vi "Pixy_COM-RIO.vi"() -> ()   [LabVIEW 2015]
uses:
  <vilib>/Analysis/baseanly.llb/Mean (DBL).vi
  <vilib>/Instr/_visa.llb/VISA Configure Serial Port (Instr).vi
  <vilib>/Analysis/NI_AALBase.lvlib
panel:
  in  "Debug?":bool
  out "Data display":string
  in  "Write Command?":bool
  in  "Command":string(combo)
  out "Area":dbl(graph)
  out "Height":i32
  out "Width":i32
  out "Y":i32
  out "X":i32
  out "Read error out":errorcluster
  out "Initialization error out":errorcluster
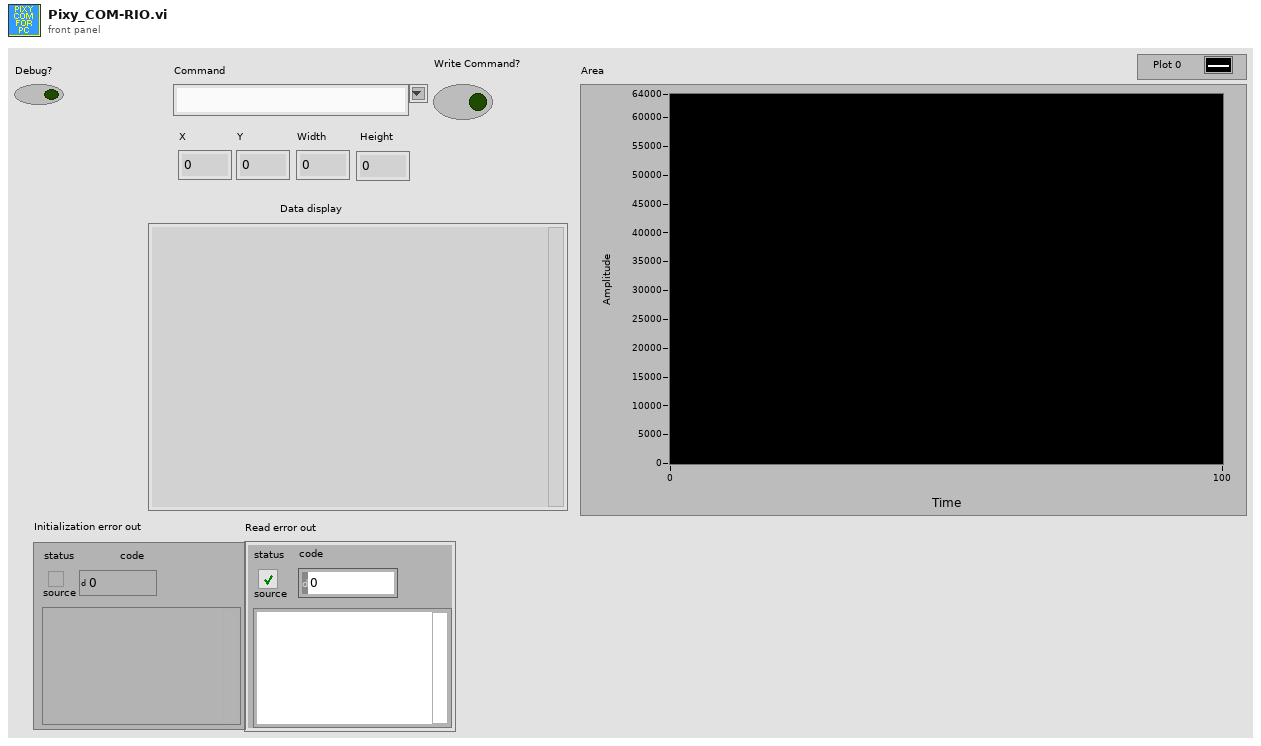
[diagram p1: front panel]
types:
  T1 = cluster{"buffer":string, "X":i32, "Y":i32, "Width":i32, "Height":i32, "Area":dbl}
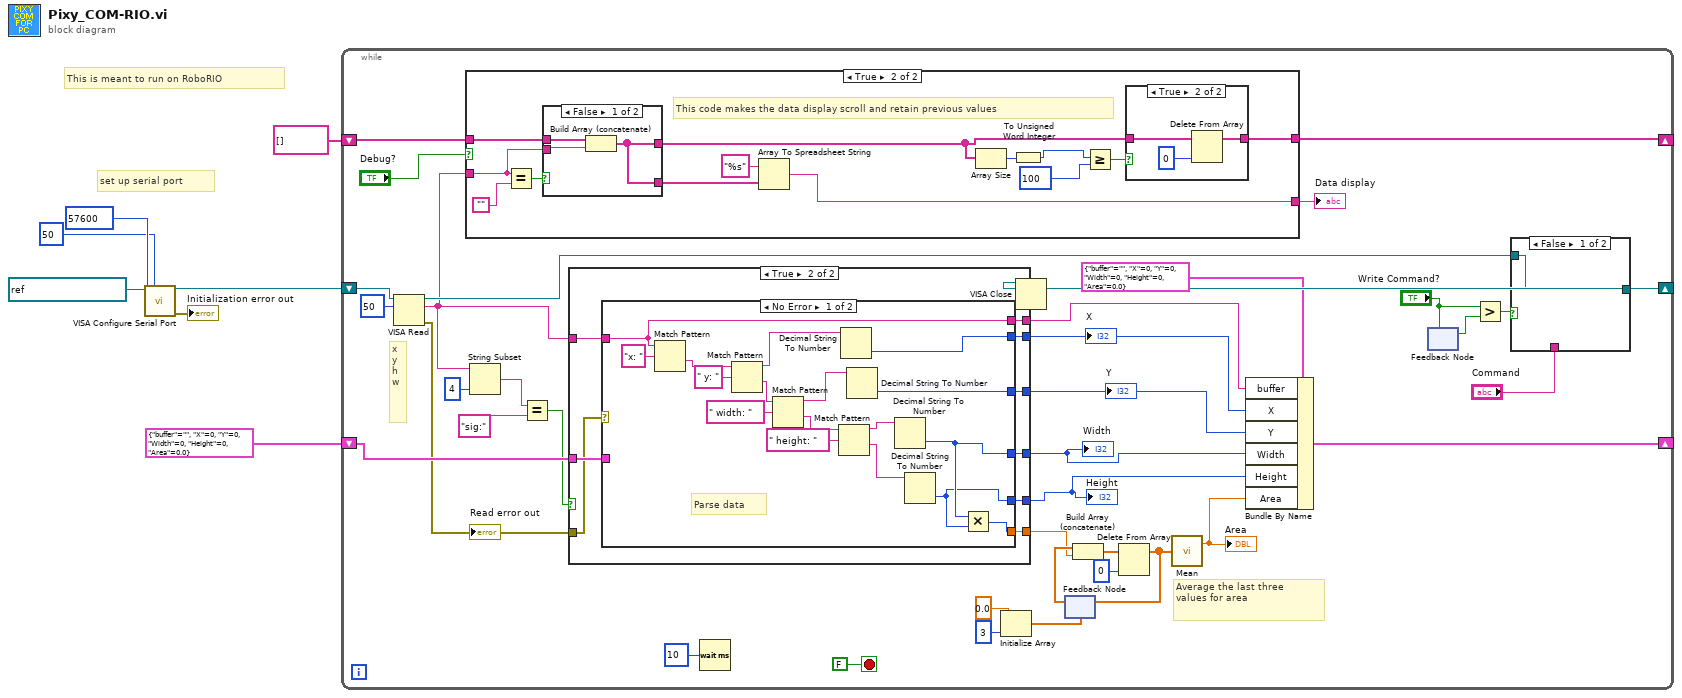
[diagram p0: block diagram]
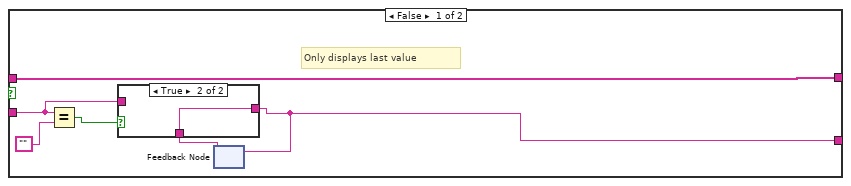
[diagram p2: hidden frame]
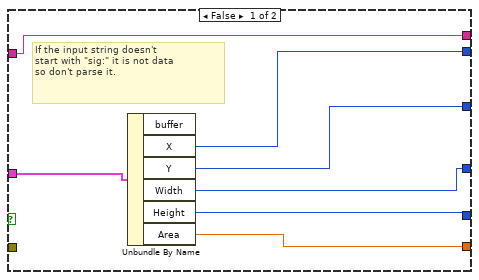
[diagram p6: hidden frame]
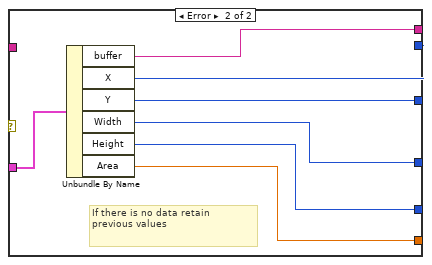
[diagram p7: hidden frame]
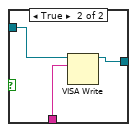
[diagram p8: hidden frame]
diagram:
  # "set up serial port"
  # "This is meant to run on RoboRIO"
  n1 = call-poly "VISA Configure Serial Port"("VISA resource name"=refnum<visa-resource-name> "ASRL3::INSTR", "timeout (10sec)"=u32 50, "baud rate (9600)"=u32 57600) -> ("VISA resource name out"=w3:refnum<visa-resource-name>, "error out"=→"Initialization error out":errorcluster)  [unwired: 11 in]
  n2 = while {
    shift-right: [w31] -> w8
    shift-left: w3 -> [w42]
    shift-right: [w41] -> _
    shift-left: T1 {"buffer"="", "X"=0, "Y"=0, "Width"=0, "Height"=0, "Area"=0.0} -> [w25]
    shift-right: [w13] -> _
    shift-left: string[] [] -> [w15]
    stop <- FALSE ("stop") stop-if-true
    # "Average the last three\nvalues for area"
    # "x\ny\nh\nw"
    n3 = VISA Read(VISA resource name=w42, byte count=u32 50) -> (VISA resource name out=w32:refnum<visa-resource-name>, read buffer=w12:string, error out=w20:errorcluster)  [unwired: 1 in, 1 out]
    "Read error out" <- w20
    n4 = case shown="True" "Debug?" {
      tunnel: w15 -> [w50 w65]
      tunnel: [w50 w61] -> w13
      tunnel: w12 -> [w48 w57]
      tunnel: [w46 w54] -> w9
      frame False {
        # "Only displays last value"
        n5 = Equal?(x=w48, y="") -> (x = y?=w49:bool)
        n6 = feedback #1() -> (w47:string)  [unwired: 1 in]
        n7 = case shown="True" w49 {
          tunnel: [w52 w53] -> w46
          tunnel: w48 -> [w52 _]
          tunnel: w47 -> [_ w53]
          frame False {
          }
          frame True {
          }
        }
        n8 = feedback-in #1(w46) -> ()
      }
      frame True {
        # "This code makes the data display scroll and retain previous values"
        n9 = Equal?(x=w57, y="") -> (x = y?=w58:bool)
        n10 = case shown="False" w58 {
          tunnel: w65 -> [w67 w70]
          tunnel: [w69 w70] -> w62
          tunnel: [w69 w70] -> w59
          tunnel: w57 -> [w68 _]
          frame False {
            n11 = Build Array (concatenate)(w67, w68) -> (w69:string[])
          }
          frame True {
          }
        }
        n12 = Array To Spreadsheet String(array=w62, 3:"%s" ("format string")) -> (spreadsheet string=w54:string)  [unwired: 1 in]
        n13 = Array Size(array=w59) -> (size(s)=w64:i32)
        n14 = To Unsigned Word Integer(number=w64) -> (unsigned 16bit integer=w63:u16)
        n15 = Greater Or Equal?(x=w63, y=u16 100 ("Display buffer size")) -> (x >= y?=w60:bool)
        n16 = case shown="True" w60 {
          tunnel: w59 -> [w71 w74]
          tunnel: [w71 w73] -> w61
          frame False {
          }
          frame True {
            n17 = Delete From Array(array=w74, index=0) -> (array with subset deleted=w73:string[])  [unwired: 1 in, 1 out]
          }
        }
      }
    }
    "Data display" <- w9
    n18 = String Subset(string=w12, length (rest)=4 ("length (rest)")) -> (substring=w21:string)  [unwired: 1 in]
    n19 = Equal?(x=w21, y="sig:") -> (x = y?=w23:bool)
    n20 = case shown="True" w23 {
      tunnel: [w75 w90] -> w30
      tunnel: [w80 w89] -> w29
      tunnel: [w79 w88] -> w28
      tunnel: [w78 w87] -> w27
      tunnel: [w77 w86] -> w11
      tunnel: [w76 w85] -> w26
      tunnel: w12 -> [w75 w84]
      tunnel: w25 -> [w81 w83]
      tunnel: w20 -> [_ w82]
      frame False {
        # "If the input string doesn't\nstart with \"sig:\" it is not data\nso don't parse it."
        n21 = Unbundle By Name(w81) -> ("X"=w80:i32, "Y"=w79:i32, "Width"=w78:i32, "Height"=w77:i32, "Area"=w76:dbl)  [unwired: 1 out]
      }
      frame True {
        n22 = case shown="No Error" w82 {
          tunnel: [w103 w109] -> w89
          tunnel: [w99 w110] -> w88
          tunnel: [w94 w111] -> w87
          tunnel: [w93 w112] -> w86
          tunnel: [w92 w113] -> w85
          tunnel: w83 -> [_ w114]
          tunnel: w84 -> [w91 _]
          tunnel: [w91 w108] -> w90
          frame No Error {
            # "Parse data"
            n23 = Match Pattern(string=w91, regular expression="x: ") -> (after substring=w106:string)  [unwired: 1 in, 3 out]
            n24 = Match Pattern(string=w106, regular expression=" y: ") -> (before substring=w104:string, after substring=w102:string)  [unwired: 1 in, 2 out]
            n25 = Match Pattern(string=w102, regular expression=" width: ") -> (before substring=w100:string, after substring=w98:string)  [unwired: 1 in, 2 out]
            n26 = Match Pattern(string=w98, regular expression=" height: ") -> (before substring=w96:string, after substring=w95:string)  [unwired: 1 in, 2 out]
            n27 = Decimal String To Number(string=w104) -> (number=w103:i32)  [unwired: 2 in, 1 out]
            n28 = Decimal String To Number(string=w100) -> (number=w99:i32)  [unwired: 2 in, 1 out]
            n29 = Decimal String To Number(string=w96) -> (number=w94:i32)  [unwired: 2 in, 1 out]
            n30 = Decimal String To Number(string=w95) -> (number=w93:i32)  [unwired: 2 in, 1 out]
            n31 = Multiply(x=w94, y=w93) -> (x*y=w92:i32)
          }
          frame Error {
            # "If there is no data retain \nprevious values"
            n32 = Unbundle By Name(w114) -> ("buffer"=w108:string, "X"=w109:i32, "Y"=w110:i32, "Width"=w111:i32, "Height"=w112:i32, "Area"=w113:dbl)
          }
        }
      }
    }
    "X" <- w29
    "Y" <- w28
    "Width" <- w27
    "Height" <- w11
    n33 = Wait (ms)(milliseconds to wait=u32 10) -> ()  [unwired: 1 out]
    n34 = Initialize Array(0.0 ("element"), 3 ("dimension size")) -> (w37:dbl[])
    n35 = feedback #2(w37) -> (w33:dbl[])
    n36 = Build Array (concatenate)(w33, w26) -> (w36:dbl[])
    n37 = Delete From Array(array=w36, index=0) -> (array with subset deleted=w35:dbl[])  [unwired: 1 in, 1 out]
    n38 = feedback-in #2(w35) -> ()
    n39 = call-poly <vilib>:"Mean.vi"("X"=w35) -> ("mean"=w40:dbl)  [unwired: 1 out]
    "Area" <- w40
    n40 = Bundle By Name(cluster=T1 {"buffer"="", "X"=0, "Y"=0, "Width"=0, "Height"=0, "Area"=0.0}, "buffer"=w30, "X"=w29, "Y"=w28, "Width"=w27, "Height"=w11, "Area"=w40) -> (w41:T1)
    n41 = feedback-in #3("Write Command?") -> ()
    n42 = feedback #3() -> (w17:bool)  [unwired: 1 in]
    n43 = Greater?(x="Write Command?", y=w17) -> (0:w18:bool)
    n44 = case shown="False" w18 {
      tunnel: w32 -> [w115 w118]
      tunnel: [w115 w117] -> w31
      tunnel: "Command" -> [_ w116]
      frame False {
      }
      frame True {
        n45 = VISA Write(VISA resource name=w118, write buffer=w116) -> (VISA resource name out=w117:refnum<visa-resource-name>)  [unwired: 1 in, 2 out]
      }
    }
  }
  n46 = VISA Close(VISA resource name=w8) -> ()  [unwired: 1 in, 1 out]
